vi "getConnectionPoint.vi"(0 "reference":refnum<class "UseCaseNode.lvclass">, 1 "direction":refnum<class "Direction.lvclass">, 5 "error in (no error)":errorcluster) -> (14 "reference out":refnum<class "UseCaseNode.lvclass">, 15 "point2D":T1 {"y" format="%.2f"; "x" format="%.2f"}, 19 "error out":errorcluster)   [LabVIEW 2016, in "UseCaseNode.lvclass"]
doc: "getConnectionPoint"
uses:
  <resource>/Framework/Providers/Open_GDS/UML/UseCaseNode_class/UseCaseNode.lvclass
  C:/Program Files (x86)/National Instruments/LabVIEW 2016/resource/Framework/Providers/Open_GDS/UML/RectangularNode_class/RectangularNode.lvclass
  <resource>/Framework/Providers/Open_GDS/UML/Direction_class/Direction.lvclass
  <resource>/Framework/Providers/Open_GDS/UML/General/Point/Point Point2D.ctl
  <resource>/Framework/Providers/Open_GDS/UML/RectangularNode_class/RectangularNode.lvclass
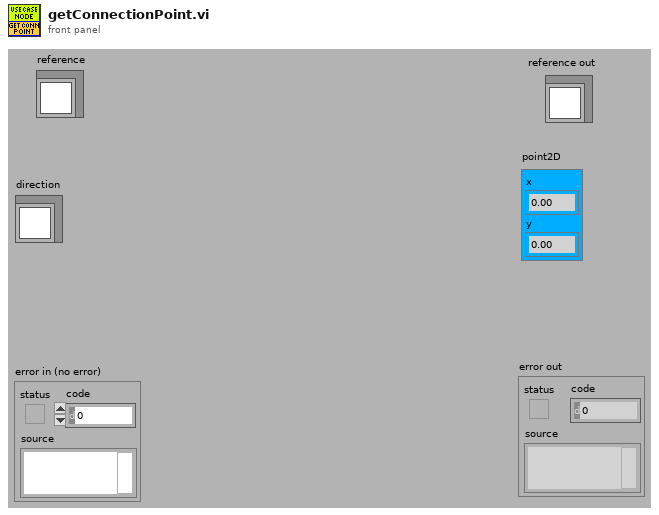
[diagram p1: front panel]
types:
  T1 = typedef "Point Point2D.ctl" = cluster{"x":dbl, "y":dbl}
  T2 = typedef "RectangularNode.lvclass/ObjectAttributes.ctl" = cluster{"bounds":T3}
  T3 = typedef "Rectangle Rectangle2D.ctl" = cluster{"x":dbl, "y":dbl, "width":dbl, "height":dbl}
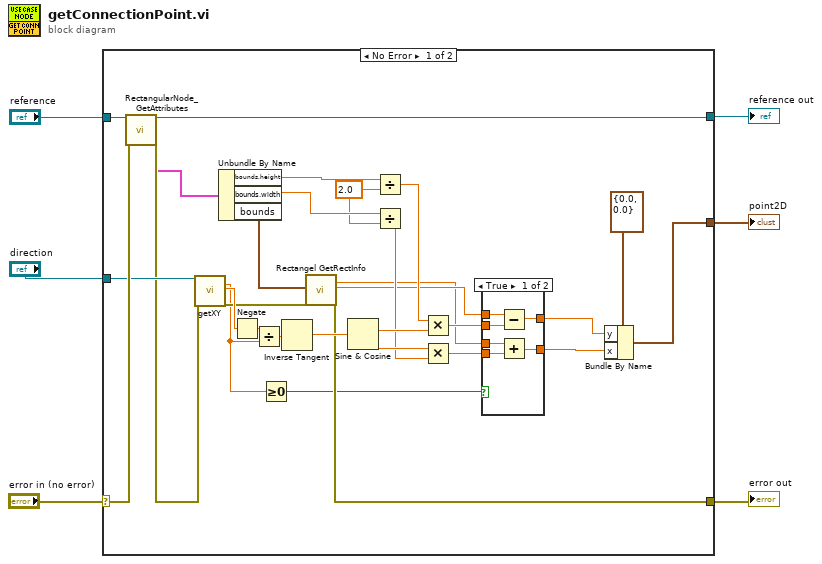
[diagram p0: block diagram]
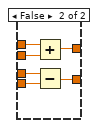
[diagram p2: hidden frame]
diagram:
  n1 = case shown="No Error" "error in (no error)" {
    selector: "error in (no error)" -> [w36 w49]
    tunnel: "reference" -> [w35 w50]
    tunnel: [w11 w49] -> w4
    tunnel: [w34 w50] -> w3
    tunnel: "direction" -> [w32 _]
    tunnel: [w12 _] -> w1
    frame No Error {
      w27 = 2.0 ("y")
      n2 = call <resource>:"RectangularNode_GetAttributes.vi"("reference in"=w35, "error in (no error)"=w36) -> ("reference out"=w34:refnum<class "UseCaseNode.lvclass">, "Data"=w7:T2, "error out"=w31:errorcluster)  [unwired: 14 in, 1 out]
      n3 = call <resource>:"getXY.vi"("reference"=w32, "error in (no error)"=w31) -> ("x"=w9:dbl, "y"=w33:dbl, "error out"=w26:errorcluster)  [unwired: 15 out]
      n4 = Unbundle By Name(w7) -> ("bounds.height"=w29:dbl, "bounds.width"=w28:dbl, "bounds"=w25:T3)
      n5 = Negate(x=w33) -> (-x=w10:dbl)
      n6 = Divide(x=w10, y=w9) -> (x/y=w30:dbl)
      n7 = Greater Or Equal To 0?(x=w9) -> (x >= 0?=w8:bool)
      n8 = Inverse Tangent(1:w30) -> (0:w24:dbl)
      n9 = call <resource>:"Rectangel GetRectInfo.vi"("bounds"=w25, "error in (no error)"=w26) -> ("centerX"=w16:dbl, "centerY"=w17:dbl, "error out"=w11:errorcluster)  [unwired: 15 out]
      n10 = Sine & Cosine(0:w24) -> (1:w22:dbl, 2:w23:dbl)
      n11 = Divide(x=w29, y=w27) -> (x/y=w21:dbl)
      n12 = Divide(x=w28, y=w27) -> (x/y=w20:dbl)
      n13 = Multiply(x=w21, y=w22) -> (x*y=w19:dbl)
      n14 = Multiply(x=w23, y=w20) -> (x*y=w18:dbl)
      n15 = case shown="True" w8 {
        tunnel: w19 -> [w42 w48]
        tunnel: w18 -> [w41 w47]
        tunnel: w17 -> [w40 w46]
        tunnel: w16 -> [w39 w45]
        tunnel: [w38 w44] -> w14
        tunnel: [w37 w43] -> w13
        frame True {
          n16 = Subtract(x=w40, y=w42) -> (x-y=w38:dbl)
          n17 = Add(x=w39, y=w41) -> (x+y=w37:dbl)
        }
        frame False {
          n18 = Add(x=w46, y=w48) -> (x+y=w44:dbl)
          n19 = Subtract(x=w45, y=w47) -> (x-y=w43:dbl)
        }
      }
      n20 = Bundle By Name(cluster=T1 {"x"=0.0, "y"=0.0} ("point2D"), "y"=w14, "x"=w13) -> (w12:T1)
    }
    frame Error {
    }
  }
  "reference out" <- w3
  "error out" <- w4
  "point2D" <- w1
